vi "Set Port Baud Rate.vi"(8 "error in":errorcluster, 10 "Baud Rate":u32, 11 "Port Ref":T1 format="%.0x") -> (0 "error out":errorcluster, 3 "Port Ref out":T1 format="%.0x")   [LabVIEW 2020, in "Communication Bus Template Scripting.lvlib"]
uses:
  <vilib>/NI VeriStand/Custom Device API/Custom Device Item Ref.ctl
  Shared/Constants.vi
  Communication Bus Template Scripting.lvlib
  <vilib>/NI VeriStand/Custom Device API/Set Item Property (U32).vi
  Shared/Communication Bus Template Shared.lvlib
  <vilib>/NI VeriStand/Custom Device API/Custom Device API.lvlib
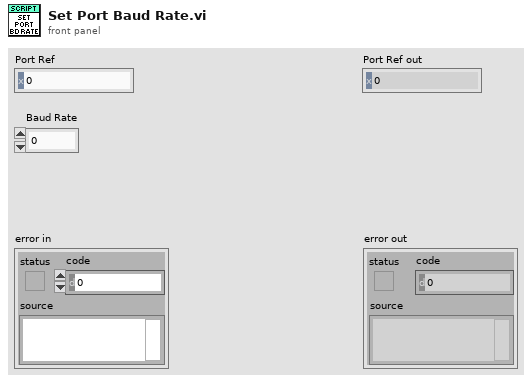
[diagram p1: front panel]
types:
  T1 = typedef "Custom Device API.lvlib/Custom Device Item Ref.ctl" = u64
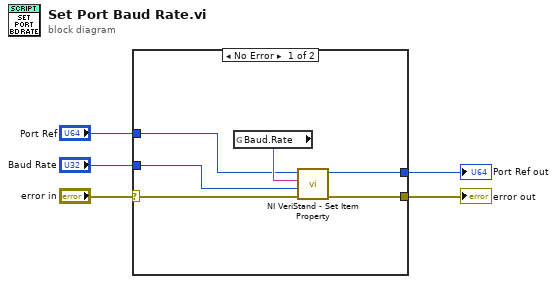
[diagram p0: block diagram]
diagram:
  n1 = case shown="No Error" "error in" {
    selector: "error in" -> [w6 w13]
    tunnel: "Port Ref" -> [w10 w12]
    tunnel: [w9 w13] -> w4
    tunnel: "Baud Rate" -> [w8 _]
    tunnel: [w7 w12] -> w2
    frame No Error {
      n2 = global read "Constants.vi" "Baud.Rate"() -> (w11:string)
      n3 = call-poly <vilib>:"NI VeriStand - Set Item Property.vi"("error in (no error)"=w6, "Value"=w8, "Property Name"=w11, "Item Ref in"=w10) -> ("error out"=w9:errorcluster, "Item Ref out"=w7:T1)  [unwired: 5 in, 1 out]
    }
    frame Error {
    }
  }
  "error out" <- w4
  "Port Ref out" <- w2
